vi "Initialize Stack Light If Enabled.vi"(8 "error in (no error)":errorcluster, 11 "DigitalIO in":refnum<class "DigitalIO.lvclass">) -> (0 "error out":errorcluster, 3 "DigitalIO out":refnum<class "DigitalIO.lvclass">)   [LabVIEW 2018, in "DigitalIO.lvlib" / "DigitalIO.lvclass"]
uses:
  DigitalIO.lvclass
  DigitalIO.lvclass/DigitalIO.ctl
  PPLs/Configuration/Configuration.lvlibp/Configuration.lvclass
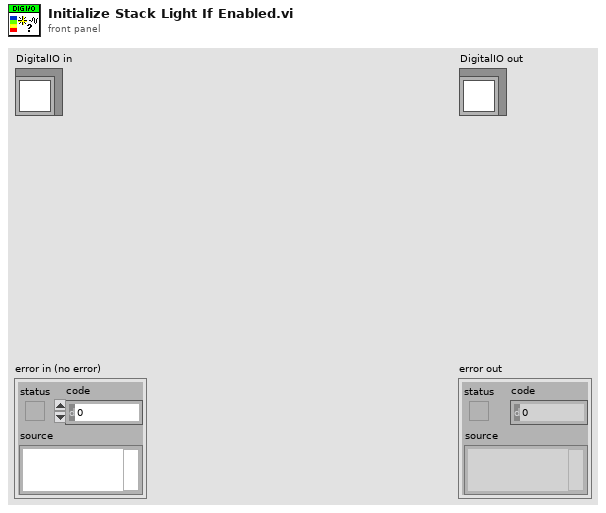
[diagram p1: front panel]
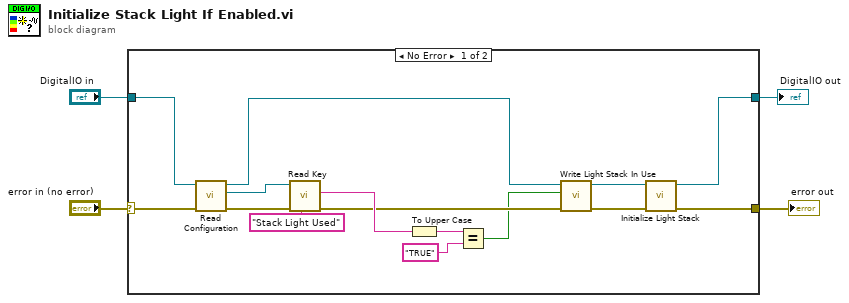
[diagram p0: block diagram]
diagram:
  n1 = case shown="No Error" "error in (no error)" {
    selector: "error in (no error)" -> [w19 w21]
    tunnel: [w5 w21] -> w3
    tunnel: [w7 w20] -> w1
    tunnel: "DigitalIO in" -> [w18 w20]
    frame No Error {
      n2 = call "Read Configuration.vi"("error in (no error)"=w19, "DigitalIO in"=w18) -> ("error out"=w16:errorcluster, "Configuration"=w17:refnum<class "Configuration.lvclass">, "DigitalIO out"=w9:refnum<class "DigitalIO.lvclass">)  [unwired: 7 in]
      n3 = call "Read Key.vi"("Key:"="Stack Light Used", "error in"=w16, "Configuration in"=w17) -> ("error out"=w11:errorcluster, "Value"=w14:string)  [unwired: 6 in, 1 out]
      n4 = To Upper Case(1:w14) -> (0:w13:string)
      n5 = Equal?(x=w13, y="TRUE") -> (x = y?=w10:bool)
      n6 = call "Write Light Stack In Use.vi"("error in (no error)"=w11, "Light Stack In Use?"=w10, "DigitalIO in"=w9) -> ("error out"=w6:errorcluster, "DigitalIO out"=w8:refnum<class "DigitalIO.lvclass">)  [unwired: 7 in]
      n7 = call "Initialize Light Stack.vi"("error in (no error)"=w6, "DigitalIO in"=w8) -> ("error out"=w5:errorcluster, "DigitalIO out"=w7:refnum<class "DigitalIO.lvclass">)  [unwired: 8 in]
    }
    frame Error {
    }
  }
  "error out" <- w3
  "DigitalIO out" <- w1
